vi "PAS IO.vi"() -> ()   [LabVIEW 2018]
uses:
  <vilib>/Platform/TimedLoop/XDataNode/timing_clust.ctl
  <vilib>/Platform/TimedLoop/XDataNode/nitl_modes.ctl
  <vilib>/Platform/TimedLoop/XDataNode/wakeup.ctl
  <vilib>/rvi/Emulation/niFpgaGetClockAttributes.vi
  <vilib>/rvi/Emulation/niFpgaSctlEmulationGetInTimedLoop.vi
  <vilib>/rvi/Emulation/niFpgaEmulationReportErrorSimple.vi
  <vilib>/rvi/Emulation/niFpgaEmulationIsFPGAContextNoSignature.vi
  <vilib>/rvi/DataTransferAndStorage/Container/Common/niFpgaContainerGetUniqueNameForEmu.vi
  <vilib>/rvi/Memory/Memory_Emulation/niFpgaMemoryEmulationCacheClearOnFirstRun.vi
  <vilib>/rvi/Memory/Memory_Emulation/nirvimemoryEmulationManagerCache_MakeExclusive.vi
  <vilib>/rvi/Memory/Memory_Emulation/niFpgaMemoryEmulationValidateCache.vi
  <vilib>/rvi/Memory/Memory_Emulation/nirvimemoryEmulationManagerCache_InsertValue.vi
  <vilib>/Utility/error.llb/Clear Errors.vi
  <vilib>/rvi/Memory/Memory_Emulation/nirvimemoryEmulationManagerCache_ReleaseExclusive.vi
  <vilib>/rvi/Memory/Memory_Emulation/nirvimemoryEmulationManagerCache_GetValue.vi
  <vilib>/rvi/Memory/Memory_Emulation/nirvimemoryEmulationManagerCache_SetValue.vi
  <vilib>/rvi/Emulation/niFpgaProcessEmulError.vi
  <vilib>/rvi/Emulation/niFpgaCriticalErrorInLSC.vi
  <vilib>/rvi/eio/common/nirviEmuTemplateMethod_errors.vi
  <vilib>/rvi/interface/RandomDataEmulation/niFpgaRandomDataHandleErrors.vi
  <vilib>/rvi/Memory/Memory_Emulation/nirvimemoryFastEmulation.vi
  <vilib>/rvi/Memory/Memory_Emulation/nirvimemoryEmulation.vi
  <vilib>/rvi/errors/nirviReportUnexpectedCaseInternalError (U32).vi
  <vilib>/rvi/DataTransferAndStorage/Container/XNode/niFpgaContainer.xnode
  <vilib>/rvi/DataTransferAndStorage/Register/Emulation/niFpgaRegisterEmulation.vi
  <vilib>/eio/EIONode/EIONode.xnode
  <vilib>/rvi/interface/RandomDataEmulation/nirviRandomDataFpgaReadWriteTemplate.vi
  <vilib>/rvi/FXPMathLib/FxpMul/XNode/nifxpmath_Multiplier.xnode
  <vilib>/rvi/FXPMathLib/FxpAdd/XNode/nifxpmath_Add.xnode
  <vilib>/Platform/TimedLoop/XDataNode/XDataNode.xnode
  <vilib>/rvi/FXPMathLib/sim/FxpSim.dll
  <vilib>/Platform/TimedLoop/XDataNode/XDNodeRunTimeDep.lvlib
panel:
  out "f1ticks":u32
  out "f0ticks":u32
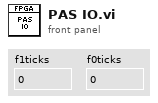
[diagram p1: front panel]
types:
  T1 = typedef "XDNodeRunTimeDep.lvlib/timing_clust.ctl" = cluster{"Expected End [f-1]":u64, "Actual End [f-1]":u64, "Finished Late? [f-1]":bool, "Expected End [i-1]":u64, "Actual End [i-1]":u64, "Finished Late? [i-1]":bool, "Expected Start [i]":u64, "Actual Start [i]":u64, "Expected Start [f]":u64, "Actual Start [f]":u64, "Source Name":string, "Structure Name":string, "Period":i64, "Deadline":i64, "Offset":i64, "Start":i64, "Priority":i32, "Timeout":i32, "Mode":T2, "Wakeup Reason":T3, "Error":errorcluster, "Source Type":string, "Secondary Source Type":string, "Global End Time":u64, "Global Start Time":u64, "Frame Duration":u64, "Iteration Duration":u64, "Assigned CPU":i32, "I/O Scan Engine Mode":u32}
  T2 = typedef "XDNodeRunTimeDep.lvlib/nitl_modes.ctl" = enum32{"No Change", "Process missed periods, maintain original phase", "Discard missed periods, maintain original phase", "Process missed periods, ignore original phase", "Discard missed periods, ignore original phase"}
  T3 = typedef "XDNodeRunTimeDep.lvlib/wakeup.ctl" = enum32{"Normal", "Aborted", "Asynchronous wakeup", "Timing source error", "Timed loop error", "Timeout"}
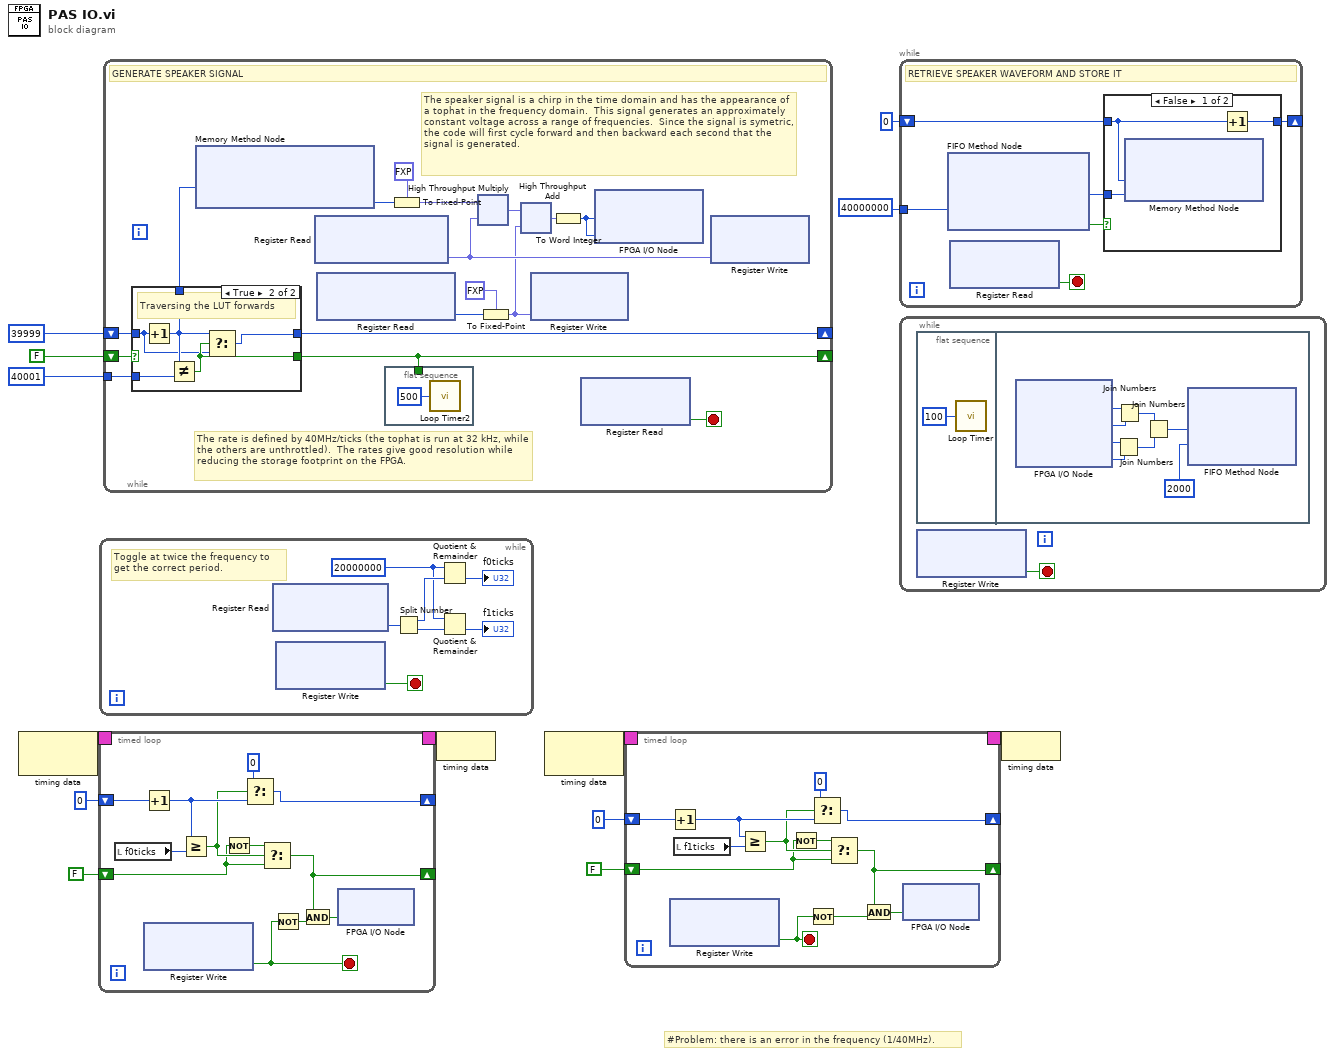
[diagram p0: block diagram]
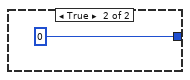
[diagram p2: hidden frame]
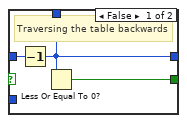
[diagram p3: hidden frame]
diagram:
  # "#Problem: there is an error in the frequency (1/40MHz)."
  n1 = node-c288() -> (w9:T1)  [unwired: 1 in]
  n2 = timed-loop {
    timing: w9 -> [_]
    timing-out: [_] -> w8
    shift-right: [w21] -> _
    shift-left: u32 0 -> [w24]
    shift-right: [w15] -> _
    shift-left: FALSE -> [w18]
    stop <- w17 stop-if-true
    n3 = local read "f0ticks"() -> (w25:u32)
    n4 = Increment(x=w24) -> (x+1=w22:u32)
    n5 = xnode ("Register Write")() -> ("Data"=w17:bool)  [unwired: 1 in, 1 out]
    n6 = Greater Or Equal?(x=w22, y=w25) -> (x >= y?=w19:bool)
    n7 = Not(x=w18) -> (.not. x?=w20:bool)
    n8 = Select(t=u32 0, s=w19, f=w22) -> (s? t:f=w21:u32)
    n9 = Select(t=w20, s=w19, f=w18) -> (s? t:f=w15:bool)
    n10 = Not(x=w17) -> (.not. x?=w16:bool)
    n11 = And(x=w15, y=w16) -> (x .and. y?=w14:bool)
    n12 = xnode "FPGA I/O Node"("PAS_1"=w14) -> ()  [unwired: 1 in, 1 out]
  }
  n13 = while {
    stop <- w34 stop-if-true
    w29 = u32 20000000 ("y")
    # "Toggle at twice the frequency to\nget the correct period."
    n14 = xnode ("Register Read")() -> ("Data"=w33:u64)  [unwired: 1 in, 1 out]
    n15 = xnode ("Register Write")() -> ("Data"=w34:bool)  [unwired: 1 in, 1 out]
    n16 = Split Number(x=w33) -> (hi(x)=w30:u32, lo(x)=w28:u32)
    n17 = Quotient & Remainder(x=w29, y=w30) -> (floor(x/y)=→"f0ticks":u32)  [unwired: 1 out]
    n18 = Quotient & Remainder(x=w29, y=w28) -> (floor(x/y)=→"f1ticks":u32)  [unwired: 1 out]
  }
  n19 = while {
    shift-right: [w46] -> _
    shift-left: FALSE -> [w51]
    shift-right: [w47] -> _
    shift-left: u32 39999 -> [w48]
    tunnel: u32 40001 ("y") -> [w49]
    stop <- w45 stop-if-true
    # "The rate is defined by 40MHz/ticks (the tophat is run at 32 kHz, while the others are unthrottled).  The rates give good resolution while reducing the storage footprint on the FPGA."
    # "The speaker signal is a chirp in the time domain and has the appearance of a tophat in the frequency domain.  This signal generates an approximately constant voltage across a range of frequencies.  Since the signal is symetric, the code will first cycle forward and then backward each second that the signal is generated."
    # "GENERATE SPEAKER SIGNAL"
    n20 = case "Check where we are in the chirp" shown="True" w51 {
      tunnel: w48 -> [w55 w56]
      tunnel: [w54 w59] -> w46
      tunnel: [w53 w60] -> w43
      tunnel: w49 -> [_ w58]
      tunnel: [w53 w57] -> w47
      frame False {
        # "Traversing the table backwards"
        n21 = Decrement(x=w55) -> (x-1=w53:u32)
        n22 = Less Or Equal To 0?(x=w53) -> (x <= 0?=w54:bool)
      }
      frame True {
        # "Traversing the LUT forwards"
        n23 = Increment(x=w56) -> (x+1=w60:u32)
        n24 = Not Equal?(x=w60, y=w58) -> (x != y?=w59:bool)
        n25 = Select(t=w60, s=w59, f=w56) -> (s? t:f=w57:u32)
      }
    }
    n26 = xnode ("Memory Method Node")("Address"=w43) -> ("Data"=w42:i16)  [unwired: 1 in, 1 out]
    n27 = xnode ("Register Read")() -> ("Data"=w38:fxp<+,32,0>)  [unwired: 1 in, 1 out]
    n28 = xnode ("Register Read")() -> ("Data"=w37:i16)  [unwired: 1 in, 1 out]
    n29 = flat-sequence {
      tunnel: w46 -> [_]
      frame #0 {
        n30 = call "Loop Timer2"("Count(Ticks)"=u32 500) -> ()  [unwired: 1 out]
      }
    }
    n31 = To Fixed-Point(fixed-point type=fxp<+/-,16,16> 0.0, number=w42) -> (fixed-point=w41:fxp<+/-,16,16>)
    n32 = xnode ("High Throughput Multiply")("x"=w41, "y"=w38) -> ("x*y"=w50:fxp<+/-,16,16>)
    n33 = To Fixed-Point(fixed-point type=fxp<+/-,16,16> 0.0, number=w37) -> (fixed-point=w36:fxp<+/-,16,16>)
    n34 = xnode ("High Throughput Add")("x"=w50, "y"=w36) -> ("x+y"=w44:fxp<+/-,16,16>)
    n35 = xnode ("Register Write")("Data"=w36) -> ()  [unwired: 1 in, 1 out]
    n36 = To Word Integer(number=w44) -> (16bit integer=w35:i16)
    n37 = xnode ("Register Read")() -> ("Data"=w45:bool)  [unwired: 1 in, 1 out]
    n38 = xnode "FPGA I/O Node"("Speaker Ch1"=w35, "Speaker Ch0"=w35) -> ()  [unwired: 2 in, 2 out]
    n39 = xnode ("Register Write")("Data"=w38) -> ()  [unwired: 1 in, 1 out]
  }
  n40 = node-c288(w8) -> ()
  n41 = node-c288() -> (w5:T1)  [unwired: 1 in]
  n42 = timed-loop {
    timing: w5 -> [_]
    timing-out: [_] -> w4
    shift-right: [w68] -> _
    shift-left: u32 0 -> [w71]
    shift-right: [w62] -> _
    shift-left: FALSE -> [w65]
    stop <- w64 stop-if-true
    n43 = Increment(x=w71) -> (x+1=w69:u32)
    n44 = xnode ("Register Write")() -> ("Data"=w64:bool)  [unwired: 1 in, 1 out]
    n45 = local read "f1ticks"() -> (w72:u32)
    n46 = Greater Or Equal?(x=w69, y=w72) -> (x >= y?=w66:bool)
    n47 = Not(x=w65) -> (.not. x?=w67:bool)
    n48 = Not(x=w64) -> (.not. x?=w63:bool)
    n49 = Select(t=u32 0, s=w66, f=w69) -> (s? t:f=w68:u32)
    n50 = Select(t=w67, s=w66, f=w65) -> (s? t:f=w62:bool)
    n51 = And(x=w62, y=w63) -> (x .and. y?=w61:bool)
    n52 = xnode "FPGA I/O Node"("PAS_2"=w61) -> ()  [unwired: 1 in, 1 out]
  }
  n53 = while {
    shift-right: [w76] -> _
    shift-left: u32 0 ("Address") -> [w77]
    tunnel: 40000000 ("Timeout") -> [w75]
    stop <- w78 stop-if-true
    # "RETRIEVE SPEAKER WAVEFORM AND STORE IT"
    n54 = xnode ("FIFO Method Node")("Timeout"=w75) -> ("Element"=w79:i16, "Timed Out?"=w80:bool)  [unwired: 1 in, 1 out]
    n55 = xnode ("Register Read")() -> ("Data"=w78:bool)  [unwired: 1 in, 1 out]
    n56 = case shown="False" w80 {
      tunnel: w79 -> [w83 _]
      tunnel: w77 -> [w81 _]
      tunnel: [w82 u32 0 ("Address")] -> w76
      frame False {
        n57 = xnode ("Memory Method Node")("Address"=w81, "Data"=w83) -> ()  [unwired: 1 in, 1 out]
        n58 = Increment(x=w81) -> (x+1=w82:u32)
      }
      frame True {
      }
    }
  }
  n59 = while {
    stop <- w85 stop-if-true
    n60 = flat-sequence {
      frame #0 {
        n61 = call "Loop Timer"("Count(uSec)"=u32 100 ("Count(Ticks)")) -> ()  [unwired: 1 out]
      }
      frame #1 {
        n62 = xnode "FPGA I/O Node"() -> ("PAS Mic 1"=w93:i16, "PAS Mic 2"=w92:i16, "PAS PD 1"=w91:i16, "PAS PD 2"=w90:i16)  [unwired: 4 in, 4 out]
        n63 = Join Numbers(hi=w91, lo=w90) -> ((hi.lo)=w88:u32)
        n64 = Join Numbers(hi=w93, lo=w92) -> ((hi.lo)=w89:u32)
        n65 = Join Numbers(hi=w89, lo=w88) -> ((hi.lo)=w87:u64)
        n66 = xnode ("FIFO Method Node")("Element"=w87, "Timeout"=2000) -> ()  [unwired: 1 in, 2 out]
      }
    }
    n67 = xnode ("Register Write")() -> ("Data"=w85:bool)  [unwired: 1 in, 1 out]
  }
  n68 = node-c288(w4) -> ()
